vi "DequeueMessage.vi"(8 "error in (no error)":errorcluster, 10 "timeout ms (-1)":i32=-1, 11 "Message Queue":refnum<queue>) -> (0 "error out":errorcluster, 1 "Message Data":variant, 2 "Message":string, 3 "dup Message Queue":refnum<queue>, 4 "timed out?":bool)   [LabVIEW 2017, in "Client.lvlib" / "CommsFrameWork.lvlib"]
doc: "This VI pulls messages off the Message Queue."
uses:
  CommsFrameWork.lvlib
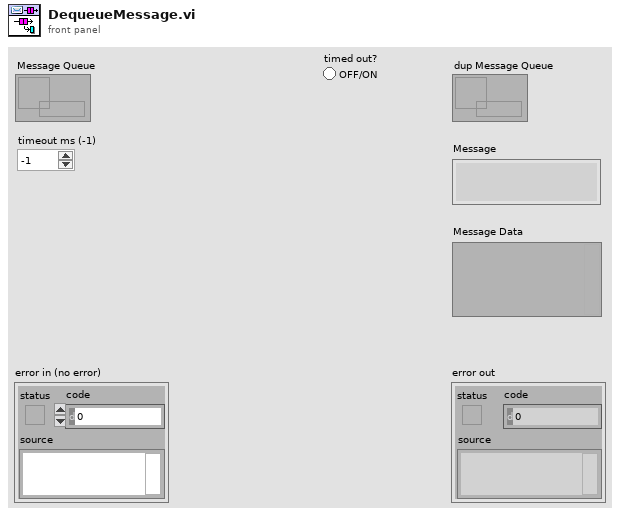
[diagram p1: front panel]
types:
  T1 = cluster{"Message":string, "Message Data":variant}
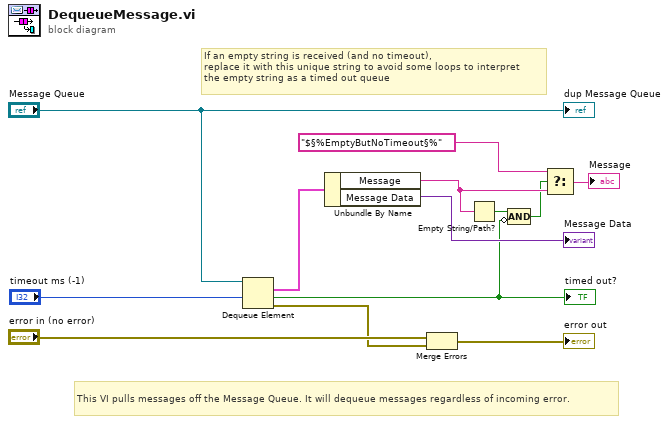
[diagram p0: block diagram]
diagram:
  # "If an empty string is received (and no timeout),\nreplace it with this unique string to avoid some loops to interpret\nthe empty string as a timed out queue"
  # "This VI pulls messages off the Message Queue. It will dequeue messages regardless of incoming error."
  n1 = Dequeue Element(queue="Message Queue", timeout in ms (-1)="timeout ms (-1)") -> (element=w11:T1, timed out?=w4:bool, error out=w8:errorcluster)  [unwired: 1 in, 1 out]
  "timed out?" <- w4
  n2 = Unbundle By Name(w11) -> ("Message"=w5:string, "Message Data"=→"Message Data":variant)
  n3 = Merge Errors("error in (no error)", w8) -> (→"error out":errorcluster)
  n4 = Empty String/Path?(string/path=w5) -> (empty?=w3:bool)
  n5 = Compound Arithmetic op=AND(w3, invert w4) -> (w2:bool)
  n6 = Select(t="$§%EmptyButNoTimeout§%", s=w2, f=w5) -> (s? t:f=→"Message":string)
  "dup Message Queue" <- "Message Queue"
